vi "getGlobalId.vi"(8 "error in (no error)":errorcluster, 11 "IComponent in":refnum<class "IComponent.lvclass">) -> (0 "error out":errorcluster, 2 "GlobalId out":string, 3 "IComponent out":refnum<class "IComponent.lvclass">)   [LabVIEW 2022 SP3, in "openDAQ.lvlib" / "IBaseObject.lvlib" / "IPropertyObject.lvlib" / "IComponent.lvlib" / "IComponent.lvclass"]
uses:
  <instrlib>/openDAQ/Public/Classes/IComponent/IComponent.lvclass
  C:/Program Files (x86)/National Instruments/LabVIEW 2022/instr.lib/openDAQ/Public/Classes/IBaseObject/IBaseObject.lvclass
  <instrlib>/openDAQ/Public/Classes/IBaseObject/IBaseObject.lvclass/IBaseObject.ctl
  <instrlib>/openDAQ/Public/Classes/IBaseObject/Accessor/Read reference.vi
  <instrlib>/openDAQ/Public/Classes/IBaseObject/Accessor/Write reference.vi
  <instrlib>/openDAQ/Public/Classes/daqCoreTypes/IString/IString.lvclass
  <instrlib>/openDAQ/Binaries/Windows/x86/copendaq32.dll
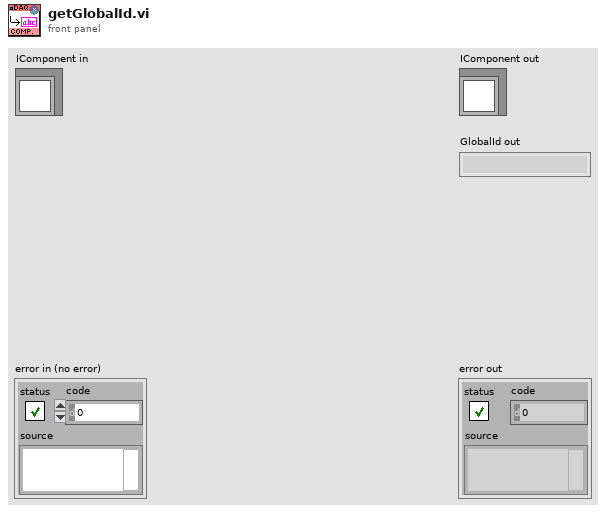
[diagram p1: front panel]
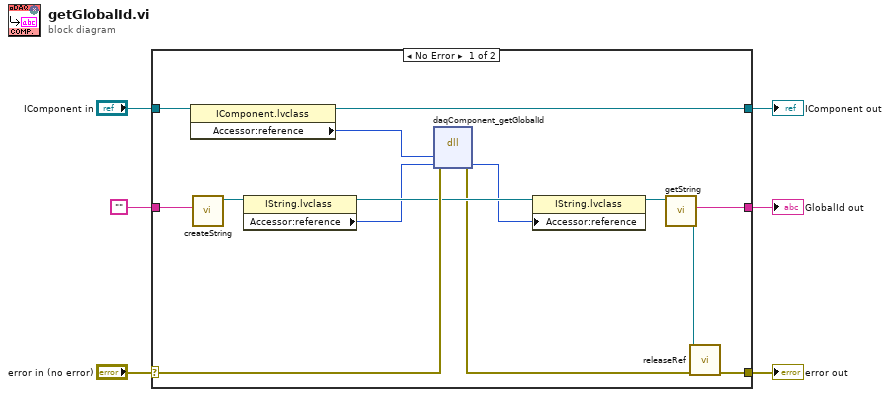
[diagram p0: block diagram]
diagram:
  n1 = case shown="No Error" "error in (no error)" {
    selector: "error in (no error)" -> [w18 w23]
    tunnel: [w9 w23] -> w5
    tunnel: [w19 w22] -> w3
    tunnel: "IComponent in" -> [w20 w22]
    tunnel: "" -> [w14 w21]
    tunnel: [w7 w21] -> w1
    frame No Error {
      n2 = property class="IComponent.lvclass"(reference=w20) -> (reference out=w19:refnum<class "IComponent.lvclass">, "Accessor:reference"=w13:i64)  [unwired: 1 in, 1 out]
      n3 = call <instrlib>:"createString.vi"("String"=w14) -> ("IString out"=w16:refnum<class "IString.lvclass">)  [unwired: 9 in, 1 out]
      n4 = property class="IString.lvclass"(reference=w16) -> (reference out=w17:refnum<class "IString.lvclass">, "Accessor:reference"=w12:i64)  [unwired: 1 in, 1 out]
      n5 = dll-call lib="C:/Program Files (x86)/National Instruments/LabVIEW 2022/instr.lib/openDAQ/Binaries/Windows/x86/copendaq*.*" fn="daqComponent_getGlobalId"(error in=w18, "component"=w13, "globalId"=w12) -> (error out=w10:errorcluster, "globalId"=w11:i64)  [unwired: 4 in, 1 out]
      n6 = property class="IString.lvclass"(reference=w17, "Accessor:reference"=w11) -> (reference out=w15:refnum<class "IString.lvclass">)  [unwired: 1 in, 1 out]
      n7 = call <instrlib>:"getString.vi"("IString in"=w15) -> ("String out"=w7:string, "IString out"=w8:refnum<class "IString.lvclass">)  [unwired: 8 in, 1 out]
      n8 = call-dynamic "releaseRef.vi"("error in (no error)"=w10, "IBaseObject in"=w8) -> ("error out"=w9:errorcluster)  [unwired: 9 in]
    }
    frame Error {
    }
  }
  "error out" <- w5
  "IComponent out" <- w3
  "GlobalId out" <- w1
